vi "发送返回状态.vi"(8 "错误输入":errorcluster, 11 "字符串":string) -> (0 "错误输出":errorcluster, 3 "返回":string)   [LabVIEW 2012]
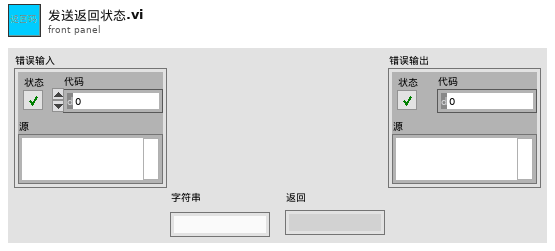
[diagram p1: front panel]
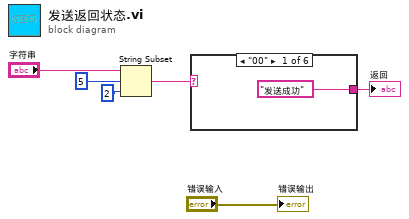
[diagram p0: block diagram]
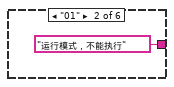
[diagram p2: hidden frame]
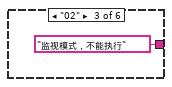
[diagram p3: hidden frame]
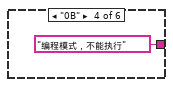
[diagram p4: hidden frame]
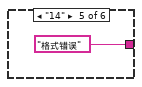
[diagram p5: hidden frame]
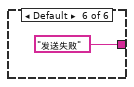
[diagram p6: hidden frame]
diagram:
  n1 = String Subset(string="字符串", offset (0)=5 ("偏移量(0)"), length (rest)=2 ("偏移量(0)")) -> (substring=w3:string)
  n2 = case shown="\"00\"" w3 {
    tunnel: ["发送成功" "运行模式，不能执行" "监视模式，不能执行" "编程模式，不能执行" "格式错误" "发送失败"] -> w2
    frame "00" {
    }
    frame "01" {
    }
    frame "02" {
    }
    frame "0B" {
    }
    frame "14" {
    }
    frame Default {
    }
  }
  "返回" <- w2
  "错误输出" <- "错误输入"
